vi "BLDC On Error.vi"() -> ()   [LabVIEW 2012, in "Phidget BLDC Motor.lvlib"]
uses:
  <instrlib>/Phidgets/Phidget BLDC Motor/Phidget BLDC Motor.lvlib
  <instrlib>/Phidgets/Phidget BLDC Motor/Public/BLDCMotorStart.vi
  <instrlib>/Phidgets/Phidget BLDC Motor/Public/BLDCMotorClose.vi
  <instrlib>/Phidgets/Phidget Common/Phidget Common.lvlib
panel:
  in  "Velocity":dbl=1.0
  in  "Stall Velocity":dbl=2000.0
  out "Serial Number Return":i32
  in  "Device Info":T1={"Serial Number"=-1, "Channel"=0, "Port"=0}
  out "error out":errorcluster
  in  "stop":bool
  out "ErrorString":string
  out "ErrorCode":i32
  # "This stall velocity is likely unreasonable\nand should cause the controller to detect\na stall even if your motor is moving freely.\nThis is to demonstrate what happens when\na stall is detected."
  # "This will receive the error generated when the motor stalls"
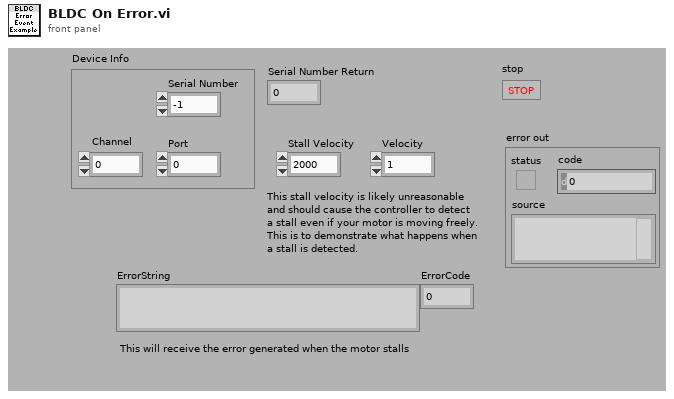
[diagram p1: front panel]
types:
  T1 = cluster{"Serial Number":i32, "Channel":i32, "Port":i32}
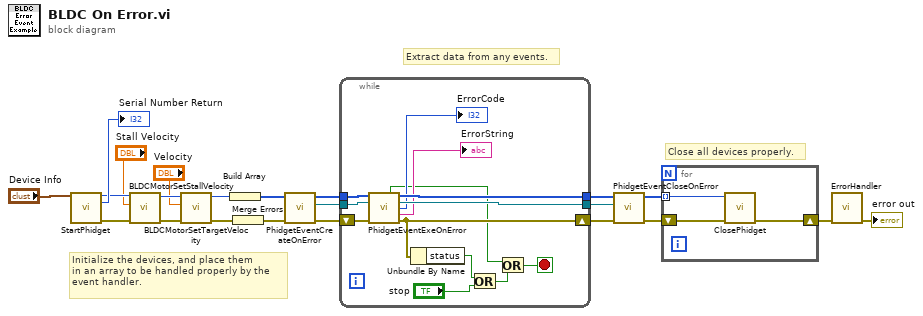
[diagram p0: block diagram]
diagram:
  # "Close all devices properly."
  # "Extract data from any events."
  # "Initialize the devices, and place them\nin an array to be handled properly by the\nevent handler."
  n1 = call-poly <instrlib>:"StartPhidget.vi"("Device Info"="Device Info") -> ("Phidget ID"=w7:u64, "Serial Number Return"=→"Serial Number Return":i32, "error out"=w8:errorcluster)  [unwired: 11 in, 1 out]
  n2 = call <instrlib>:"BLDCMotorSetStallVelocity.vi"("error in (no error)"=w8, "Stall Velocity"="Stall Velocity", "Device In"=w7) -> ("error out"=w5:errorcluster, "Device Out"=w6:u64)  [unwired: 6 in]
  n3 = call <instrlib>:"BLDCMotorSetTargetVelocity.vi"("error in (no error)"=w5, "Velocity"="Velocity", "Device In"=w6) -> ("error out"=w4:errorcluster, "Device Out"=w3:u64)  [unwired: 6 in]
  n4 = Build Array(w3) -> (w22:u64[])
  n5 = Merge Errors(w4) -> (w13:errorcluster)
  n6 = call <instrlib>:"PhidgetEventCreateOnError.vi"("error in (no error)"=w13, "Devices In"=w22) -> ("error out"=w15:errorcluster, "Event Registration Refnum"=w20:refnum<event-registration>, "Devices Out"=w21:u64[])  [unwired: 7 in]
  n7 = while {
    tunnel: w21 -> [w35]
    tunnel: w20 -> [w32]
    tunnel: [w34] -> w17
    shift-right: [w26] -> w16
    shift-left: w15 -> [w33]
    tunnel: [w29] -> w10
    stop <- w24 stop-if-true
    n8 = call <instrlib>:"PhidgetEventExeOnError.vi"("Devices In"=w35, "Event Registration Refnum In"=w32, "error in (no error)"=w33) -> ("Event?"=w23:bool, "Devices Out"=w29:u64[], "Event Registration Refnum Out"=w34:refnum<event-registration>, "ErrorCode"=→"ErrorCode":i32, "ErrorString"=→"ErrorString":string, "error out"=w26:errorcluster)  [unwired: 5 in, 2 out]
    n9 = Unbundle By Name(w26) -> ("status"=w30:bool)
    n10 = Or(x=w30, y="stop") -> (x .or. y?=w25:bool)
    n11 = Or(x=w23, y=w25) -> (x .or. y?=w24:bool)
  }
  n12 = call <instrlib>:"PhidgetEventCloseOnError.vi"("error in (no error)"=w16, "Event Registration Refnum In"=w17, "Devices In"=w10) -> ("error out"=w12:errorcluster, "Devices Out"=w11:u64[])  [unwired: 7 in]
  n13 = for {
    tunnel: w11 -> [w36] mode=indexing
    shift-right: [w38] -> w19
    shift-left: w12 -> [w37]
    n14 = call-poly <instrlib>:"ClosePhidget.vi"("error in"=w37, "Device In"=w36) -> ("error out"=w38:errorcluster)  [unwired: 9 in]
  }
  n15 = call <instrlib>:"ErrorHandler.vi"("error in"=w19) -> ("error out"=→"error out":errorcluster)  [unwired: 9 in, 1 out]
